vi "WriteByteArray.vi"(4 "Input":u8[](array[numeric]), 6 "Address Areas":T2=132 items=["Input(I)"=129, "Output(Q)"=130, "Bit Memory(M)"=131, "Data(DB)"=132], 7 "Bit/Byte":u8(ring)=2 items=["Boolen"=1, "Byte"=2], 8 "error in (no error)":errorcluster, 9 "Offset":u16, 10 "#DB No.":u16, 11 "Siemens Ctr in":T1) -> (0 "error out (no error)":errorcluster, 1 "Error message":string, 2 "Data valid?":bool, 3 "Siemens Ctr out":T1)   [LabVIEW 2014, in "Simatic S7.lvlib"]
uses:
  Simatic S7.lvlib
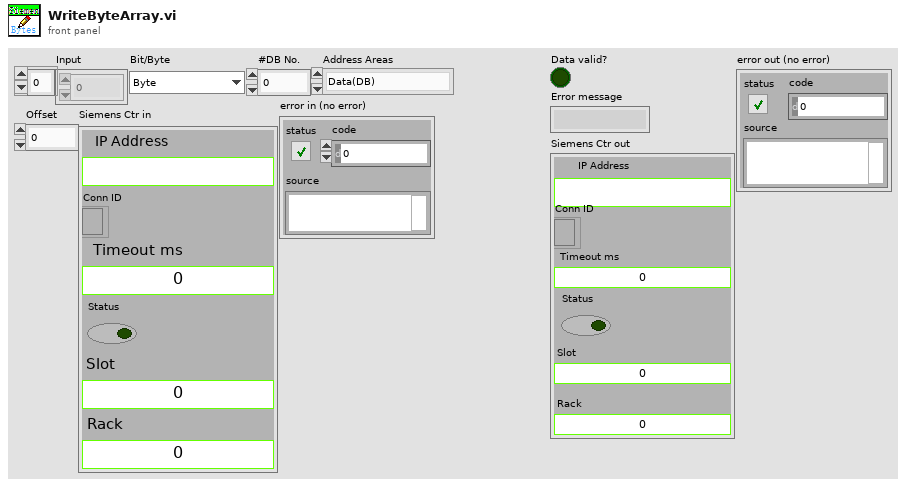
[diagram p1: front panel]
types:
  T1 = typedef "Simatic S7.lvlib/Siemens Ref.ctl" = cluster{"IP Address ":string, "Conn ID":refnum<k5>, "Timeout ms":i32, "Status":bool, "Slot":u16, "Rack":u16}
  T2 = typedef "Simatic S7.lvlib/Address Areas.ctl" = u8
  T3 = typedef "Data Type.ctl" = enum8{"Bit", "Byte (U8)", "Signed Byte (I8)", "Word (U16)", "Signed Word (I16)", "Long (U32)", "Signed Long (I32)", "Real (SGL)", "String"}
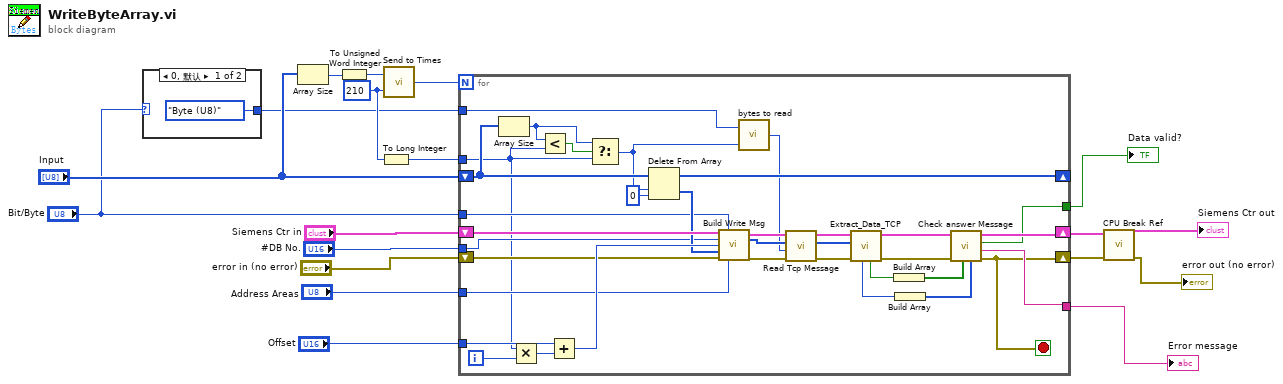
[diagram p0: block diagram]
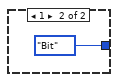
[diagram p2: hidden frame]
diagram:
  w15 = u8 210 ("max items per request")
  n1 = case shown="0, 默认" "Bit/Byte" {
    tunnel: [Data_Type."Byte (U8)" ("Data Type") Data_Type."Bit" ("Data Type")] -> w7
    frame 0, Default {
    }
    frame 1 {
    }
  }
  n2 = Array Size(array="Input") -> (size(s)=w17:i32)
  n3 = To Unsigned Word Integer(number=w17) -> (unsigned 16bit integer=w18:u16)
  n4 = To Long Integer(number=w15) -> (32bit integer=w14:i32)
  n5 = call "Send to Times.vi"("max items per request"=w15, "#items"=w18) -> ("for loop request"=w19:u16)
  n6 = for {
    N: w19 -> [_]
    shift-right: [w46] -> _
    shift-left: "Input" -> [w49]
    tunnel: w14 -> [w23]
    tunnel: "Offset" -> [w52]
    shift-right: [w27] -> w3
    shift-left: "Siemens Ctr in" -> [w50]
    tunnel: "Bit/Byte" -> [w41]
    tunnel: "#DB No." -> [w45]
    shift-right: [w22] -> w4
    shift-left: "error in (no error)" -> [w44]
    tunnel: "Address Areas" -> [w43]
    tunnel: w7 -> [w40]
    tunnel: [w26] -> w6
    tunnel: [w25] -> w5
    i -> [w54]
    stop <- w22 stop-if-true
    n7 = Array Size(array=w49) -> (size(s)=w55:i32)
    n8 = Multiply(x=w23, y=w54) -> (x*y=w53:i32)
    n9 = Less?(x=w55, y=w23) -> (x < y?=w56:bool)
    n10 = Add(x=w52, y=w53) -> (x+y=w51:i32)
    n11 = Select(t=w55, s=w56, f=w23) -> (s? t:f=w42:i32)
    n12 = Delete From Array(array=w49, length=w42, index=0) -> (deleted portion=w47:u8[], array with subset deleted=w46:u8[])
    n13 = call "Build Write Msg.vi"("Siemens Ctr in"=w50, "Bit/Byte"=w41, "#DB No."=w45, "#offset"=w51, "Input"=w47, "error in (no error)"=w44, "Address Areas"=w43) -> ("Siemens Ctr out"=w38:T1, "appended array"=w37:u8[], "error out"=w39:errorcluster)  [unwired: 6 in]
    n14 = call "bytes to read.vi"("Items"=w42, "Data Type"=w40) -> ("Bytes to read"=w36:i32)
    n15 = call "Read Tcp Message.vi"("error in (no error)"=w39, "bytes to read"=w36, "Request Message"=w37, "Siemens Ctr"=w38) -> ("error out"=w35:errorcluster, "Recieve Message"=w24:u8[], "S7 Connection out"=w34:T1)  [unwired: 4 in, 1 out]
    n16 = call "Extract_Data_TCP.vi"("error in (no error)"=w35, "Data Recieved"=w24, "Siemens Ctr in"=w34) -> ("error out"=w32:errorcluster, "Siemens Ctr"=w33:T1, "Data Valid"=w31:bool, "Error Code"=w29:u8)  [unwired: 2 in, 3 out]
    n17 = Build Array(w31) -> (w30:bool[])
    n18 = Build Array(w29) -> (w28:u8[])
    n19 = call "Check answer Message.vi"("Error id"=w28, "data valid?"=w30, "error in (no error)"=w32, "Siemens Ctr"=w33) -> ("error out"=w22:errorcluster, "Error message"=w25:string, "Data valid?"=w26:bool, "Siemens Ctr out"=w27:T1)  [unwired: 4 in]
  }
  "Data valid?" <- w6
  "Error message" <- w5
  n20 = call "CPU Break Ref.vi"("error in (no error)"=w4, "Siemens Ctr"=w3) -> ("error out"=→"error out (no error)":errorcluster, "Siemens Ctr out"=→"Siemens Ctr out":T1)  [unwired: 8 in]
